vi "ThresholdBinary.vi"(4 "Max Value (Default: 255)":u8=255, 6 "Invert? (Default: False)":bool, 7 "Threshold":u8, 8 "error in (no error)":errorcluster, 10 "Threshold Result":refnum<data-value>, 11 "Greyscale Image-Source":refnum<data-value>) -> (0 "error out":errorcluster, 3 "Threshold Result (duplicate)":refnum<data-value>)   [LabVIEW 2020, in "g_ar_toolkit.image.lvlib"]
uses:
  g_ar_toolkit.image.lvlib
  Threshold Types.ctl
  g_ar_toolkit.common/Module Path.vi
  <vilib>/Utility/error.llb/Error Cluster From Error Code.vi
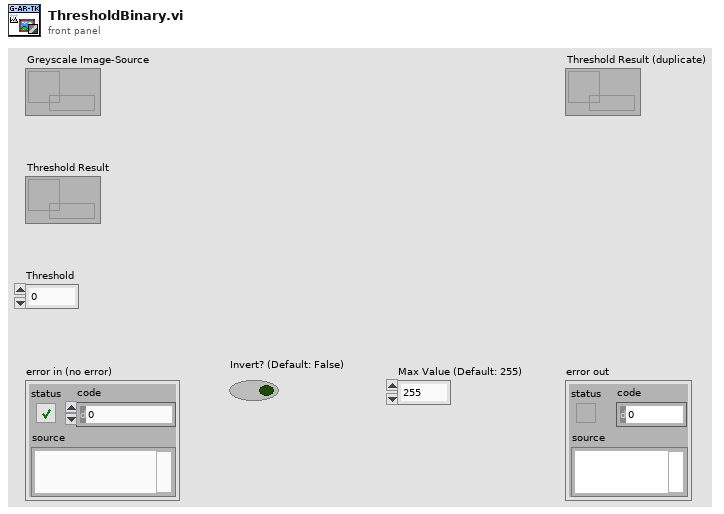
[diagram p1: front panel]
types:
  T1 = typedef "g_ar_toolkit.image.lvlib/Threshold Types.ctl" = enum8{"THRESH_BINARY", "THRESH_BINARY_INV", "THRESH_TRUNC", "THRESH_TOZERO", "THRESH_TOZERO_INV", "THRESH_MASK", "THRESH_OTSU", "THRESH_TRIANGLE"}
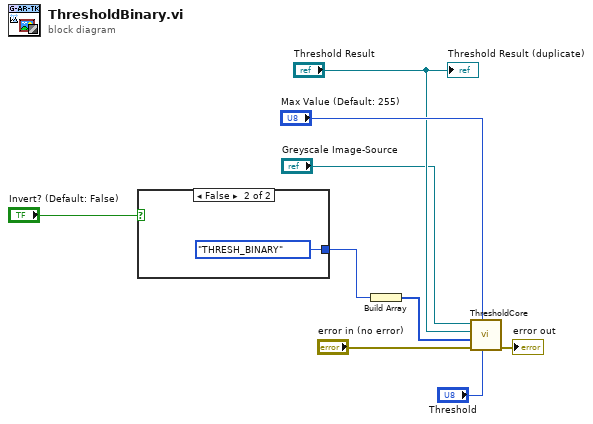
[diagram p0: block diagram]
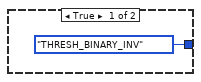
[diagram p2: hidden frame]
diagram:
  n1 = case shown="False" "Invert? (Default: False)" {
    tunnel: [Threshold_Types."THRESH_BINARY_INV" ("Threshold Types") Threshold_Types."THRESH_BINARY" ("Threshold Types")] -> w2
    frame True {
    }
    frame False {
    }
  }
  n2 = Build Array(w2) -> (w1:T1[])
  n3 = call "ThresholdCore.vi"("Threshold"="Threshold", "Max Value"="Max Value (Default: 255)", "error in (no error)"="error in (no error)", "Mode"=w1, "Threshold Result"="Threshold Result", "Greyscale Image-Source"="Greyscale Image-Source") -> ("error out"=→"error out":errorcluster)  [unwired: 5 in]
  "Threshold Result (duplicate)" <- "Threshold Result"
